vi "Update Data.vi"(8 "error in":errorcluster, 10 "output cluster":T1) -> (0 "error out":errorcluster)   [LabVIEW 2024, in "UIs Handler.lvlib"]
doc: "Update Data\n\n_____\nCreated using DQMH Framework: Event Scripter 7.1.0.1490."
uses:
  UIs Handler.lvlib
  Update Data Argument--cluster.ctl
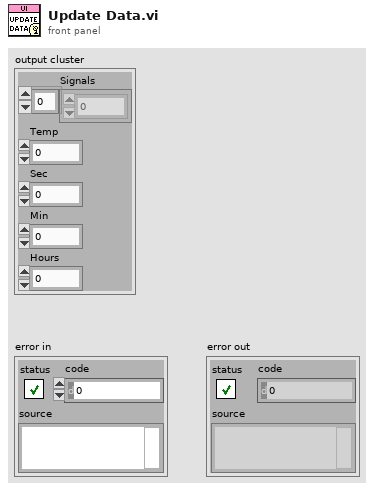
[diagram p1: front panel]
types:
  T1 = cluster{"Signals":dbl[], "Temp":dbl, "Sec":i32, "Min":i32, "Hours":i32}
  T2 = typedef "UIs Handler.lvlib/Update Data Argument--cluster.ctl" = cluster{"output cluster":cluster{"Signals":dbl[], "Temp":dbl, "Sec":i32, "Min":i32, "Hours":i32}}
  T3 = typedef "UIs Handler.lvlib/Broadcast Events--cluster.ctl" = cluster{"Module Did Init":refnum<user-event>, "Status Updated":refnum<user-event>, "Error Reported":refnum<user-event>, "Module Did Stop":refnum<user-event>, "Update Module Execution Status":refnum<user-event>, "Update Data":refnum<user-event>}
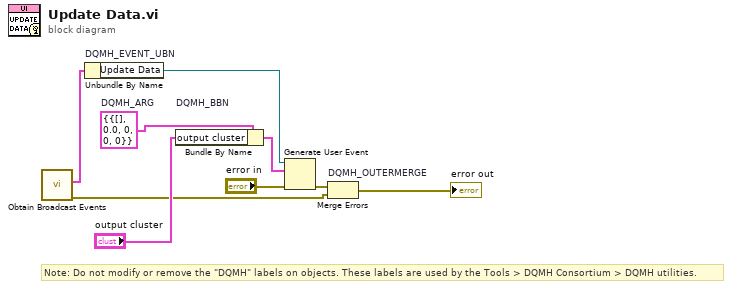
[diagram p0: block diagram]
diagram:
  w4 = T2 {"output cluster"={"Signals"=[], "Temp"=0.0, "Sec"=0, "Min"=0, "Hours"=0}}  # DQMH_ARG
  # "Note: Do not modify or remove the \"DQMH\" labels on objects. These labels are used by the Tools > DQMH Consortium > DQMH utilities."
  n1 = call "Obtain Broadcast Events.vi"() -> ("error out"=w2:errorcluster, "UIs Handler Broadcast Events"=w1:T3)  [unwired: 10 in]
  n2 = Unbundle By Name "DQMH_EVENT_UBN"(w1) -> ("Update Data"=w6:refnum<user-event>)
  n3 = Bundle By Name "DQMH_BBN"(cluster=w4, "output cluster"="output cluster") -> (w7:T2)
  n4 = Generate User Event(user event=w6, event data cluster=w7, error in="error in") -> (error out=w5:errorcluster)  [unwired: 1 in, 1 out]
  n5 = Merge Errors "DQMH_OUTERMERGE"(w5, w2) -> (→"error out":errorcluster)
